vi "Hooks Search Path.vi"(1 "Additional Search Path":path[](array[path])) -> (0 "Hooks Search Path":path[](array[path]))   [LabVIEW 2018, in "Toolkit.lvlib"]
uses:
  Toolkit.lvlib
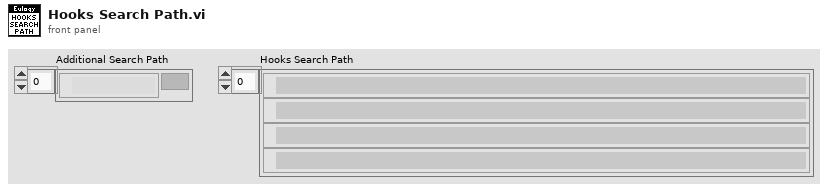
[diagram p1: front panel]
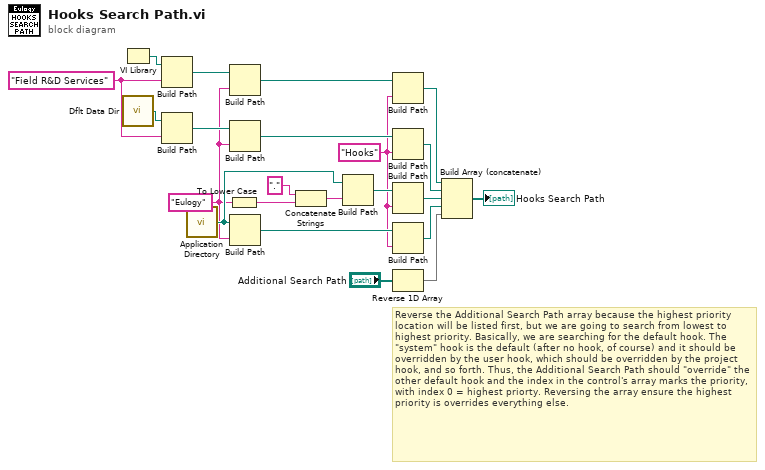
[diagram p0: block diagram]
diagram:
  w6 = "Hooks" ("name or relative path")
  w1 = "Eulogy" ("name or relative path")
  w18 = "Field R&D Services" ("name or relative path")
  # "Reverse the Additional Search Path array because the highest priority location will be listed first, but we are going to search from lowest to highest priority. Basically, we are searching for the default hook. The \"system\" hook is the default (after no hook, of course) and it should be overridden by the user hook, which should be overridden by the project hook, and so forth. Thus, the Additional Search Path should \"override\" the other default hook and the index in the control's array marks the priority, with index 0 = highest priorty. Reversing the array ensure the highest priority is overrides everything else."
  n1 = VI Library() -> (path=w22:path)
  n2 = call <vilib>:"Dflt Data Dir.vi"() -> ("App:Default Data Directory"=w19:path)
  n3 = Build Path(base path=w22, name or relative path=w18) -> (appended path=w21:path)
  n4 = Build Path(base path=w19, name or relative path=w18) -> (appended path=w17:path)
  n5 = call <vilib>:"Application Directory.vi"() -> ("Application Directory"=w8:path)
  n6 = To Lower Case(string=w1) -> (all lower case string=w4:string)
  n7 = Build Path(base path=w21, name or relative path=w1) -> (appended path=w20:path)
  n8 = Build Path(base path=w17, name or relative path=w1) -> (appended path=w16:path)
  n9 = Build Path(base path=w8, name or relative path=w1) -> (appended path=w7:path)
  n10 = Concatenate Strings("." ("string"), w4) -> (w2:string)
  n11 = Build Path(base path=w8, name or relative path=w2) -> (appended path=w13:path)
  n12 = Build Path(base path=w20, name or relative path=w6) -> (appended path=w15:path)
  n13 = Build Path(base path=w16, name or relative path=w6) -> (appended path=w14:path)
  n14 = Build Path(base path=w13, name or relative path=w6) -> (appended path=w12:path)
  n15 = Build Path(base path=w7, name or relative path=w6) -> (appended path=w5:path)
  n16 = Reverse 1D Array(array="Additional Search Path") -> (reversed array=w9:path[])
  n17 = Build Array (concatenate)(w15, w14, w12, w5, w9) -> (→"Hooks Search Path":path[])
